vi "View TDMS.vi"() -> ()   [LabVIEW 2021]
uses:
  <vilib>/Utility/TDMS File Viewer/TDMS - File Viewer (NXG Style).vi
  <vilib>/Utility/TDMS File Viewer/NI_TDMS File Viewer.lvlib
panel:
  out "error out":errorcluster
  out "application name":string
  out "Arguments":string[](array[string])
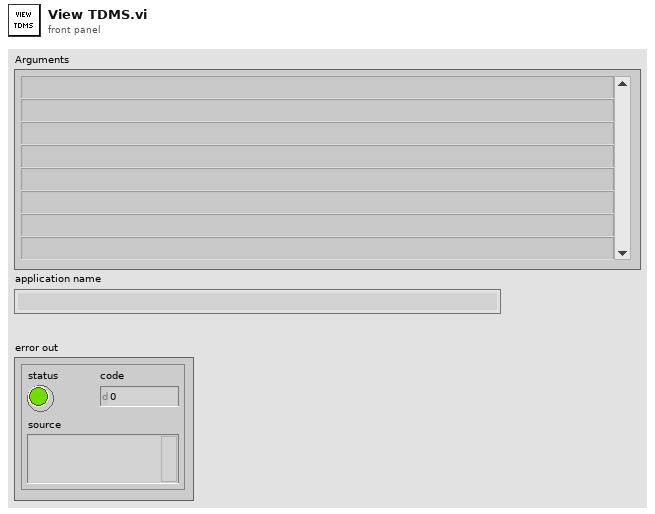
[diagram p1: front panel]
types:
  T1 = enum32{"Invalid", "Standard", "Closed", "Hidden", "Minimized", "Maximized"}
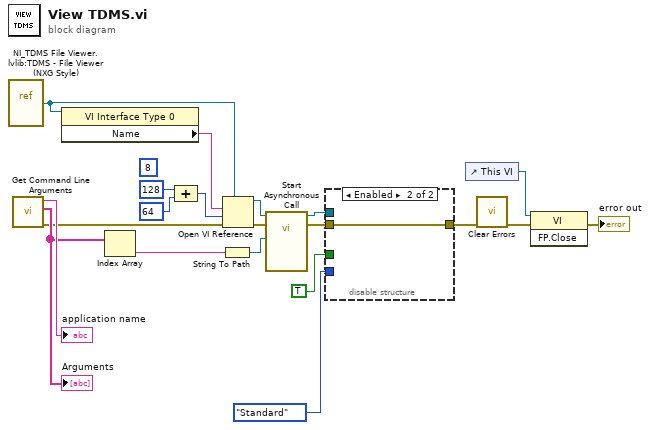
[diagram p0: block diagram]
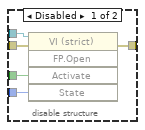
[diagram p2: hidden frame]
diagram:
  (unwired) 8 ("options")
  n1 = vi-ref "NI_TDMS File Viewer.lvlib:TDMS - File Viewer (NXG Style).vi"() -> (w8:refnum<vi>)
  n2 = call <vilib>:"Get Command Line Arguments.vi"() -> ("error out"=w6:errorcluster, "arguments"=w19:string[], "application name"=→"application name":string)  [unwired: 9 in]
  "Arguments" <- w19
  n3 = property class="VI Interface Type 0"(reference=w8) -> ("Name"=w7:string)  [unwired: 1 in, 2 out]
  n4 = Index Array(array=w19) -> (element=w18:string)  [unwired: 1 in]
  n5 = Compound Arithmetic op=unknown(128 ("options"), 64 ("options")) -> (w1:i32)
  n6 = String To Path(string=w18) -> (path=w14:path)
  n7 = Open VI Reference(type specifier VI Refnum (for type only)=w8, vi path=w7, options=w1, error in (no error)=w6) -> (vi reference=w4:refnum<vi>, error out=w5:errorcluster)  [unwired: 2 in]
  n8 = call-by-ref "Start Asynchronous Call"(reference=w4, error in=w5, "file in"=w14) -> (reference out=w11:refnum<vi>, error out=w13:errorcluster)  [unwired: 9 in, 2 out]
  n9 = disable-structure shown="Enabled" {
    disable-tunnel: w13 -> [w25 w26]
    disable-tunnel: [w24 w26] -> w12
    disable-tunnel: w11 -> [w23 _]
    disable-tunnel: TRUE ("Activate?") -> [w22 _]
    disable-tunnel: T1."Standard" ("State") -> [w21 _]
    frame Disabled {
      n10 = invoke class="VI (strict)" method="FP.Open"(reference=w23, error in=w25, "Activate"=w22, "State"=w21) -> (error out=w24:errorcluster)  [unwired: 1 in, 4 out]
    }
    frame Enabled {
    }
  }
  n11 = control-ref of="This VI"() -> (w17:refnum<vi>)
  n12 = call <vilib>:"Clear Errors.vi"("error in (no error)"=w12) -> ("error out"=w16:errorcluster)  [unwired: 5 in, 1 out]
  n13 = invoke class="VI" method="FP.Close"(reference=w17, error in=w16) -> (error out=→"error out":errorcluster)  [unwired: 1 in, 2 out]
